vi "Init.vi"(5 "PathControl.lvclass":refnum<class "PathControl.lvclass">, 6 "Environmental classes":refnum<class "Instrument.lvclass">[](array[class]), 7 "XML Handler.lvclass":refnum<class "XML Handler.lvclass">, 8 "error in (no error)":errorcluster, 9 "Instrumentes to Use":T2(array[cluster]), 10 "Device.lvclass":refnum<class "Device.lvclass">, 11 "S Parameter in":refnum<class "S Parameter.lvclass">) -> (0 "error out":errorcluster, 3 "S Parameter out":refnum<class "S Parameter.lvclass">)   [LabVIEW 2020, in "S Parameter.lvclass"]
doc: "Initializes the measurement.\nThis verifies that the instruments are present and adds them into the class data.\nIs also adds the xml handler into the class data."
uses:
  S Parameter.lvclass
  Devices/Device.lvclass
  Instruments/Instrument.lvclass
  XML Handler/XML Handler.lvclass
  Path Control/PathControl.lvclass
  Controls/Init State Machine.ctl
  Instruments/Vector Network Analyzer/Vector Network Analyzer.lvclass
  S Parameter.lvclass/S Parameter.ctl
  Instruments/Vector Network Analyzer/Controls/S parm format enum.ctl
  Measurement.lvclass
panel:
  in  "S parameter":T1(ring)
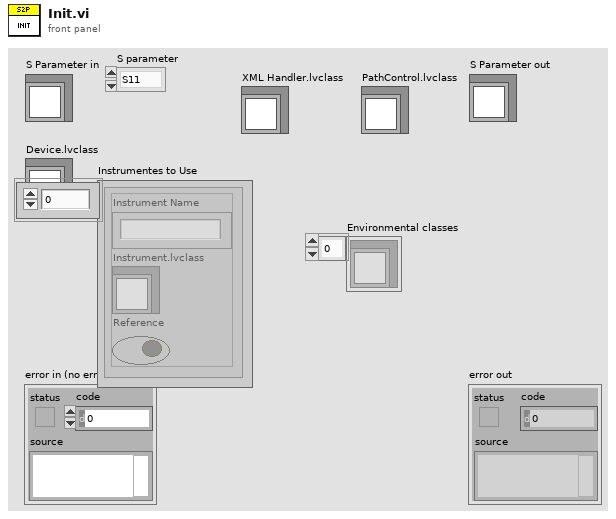
[diagram p1: front panel]
types:
  T1 = enum16{"S11", "S21", "S31", "S41", "S22", "S12", "S32", "S42", "S33", "S13", "S23", "S43", "S44", "S14", "S24", "S34"}
  T2 = cluster{"Instrument Name":string, "Instrument.lvclass":refnum<class "Instrument.lvclass">, "Reference":bool}[]
  T3 = typedef "S Parameter.lvclass/Init State Machine.ctl" = enum16{"Verify Instruments", "Init Instruments", "Init Device", "Create test in XML", "Set Path", "Done"}
  T4 = typedef "Vector Network Analyzer.lvclass/S parm format enum.ctl" = enum16{"Mag dB", "Mag", "Phase", "Smith", "Real", "Imag", "Group Delay", "SWR"}
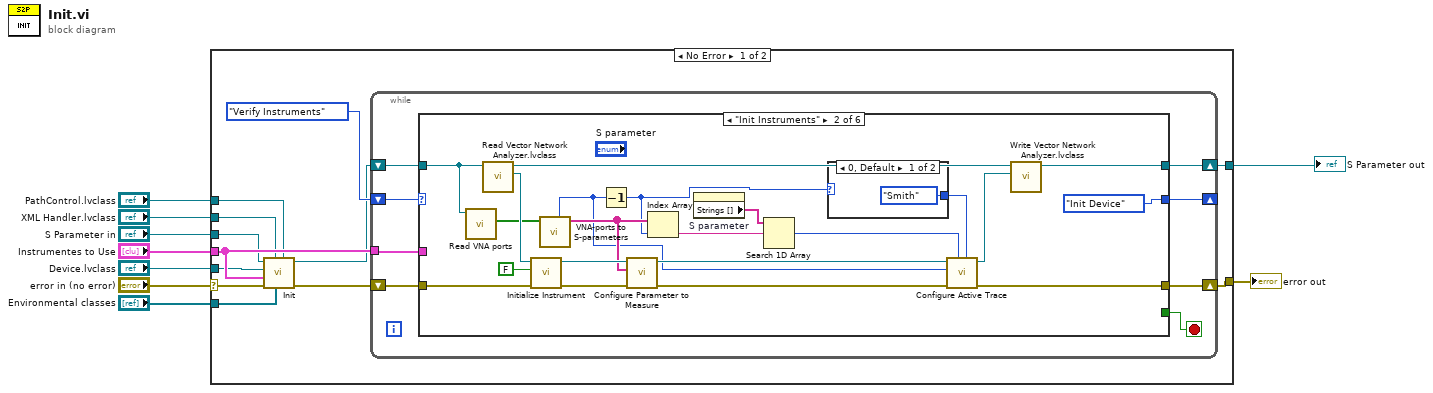
[diagram p0: block diagram]
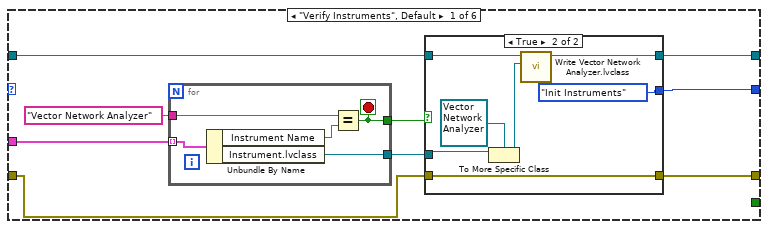
[diagram p2: hidden frame]
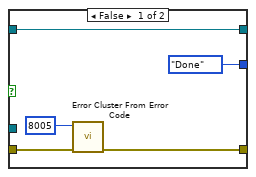
[diagram p3: hidden frame]
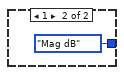
[diagram p4: hidden frame]
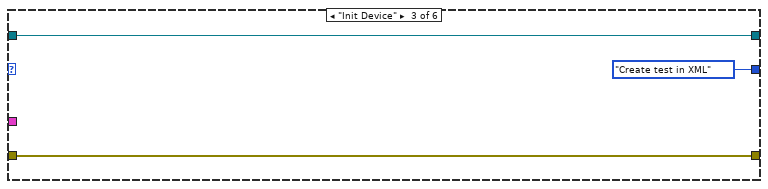
[diagram p5: hidden frame]
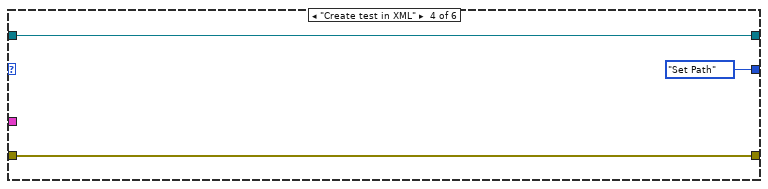
[diagram p6: hidden frame]
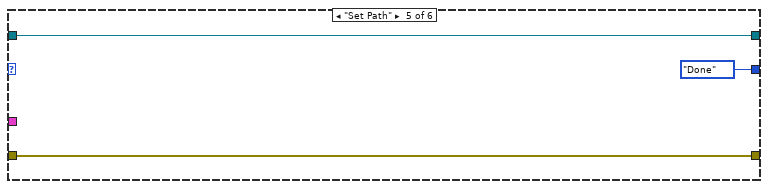
[diagram p7: hidden frame]
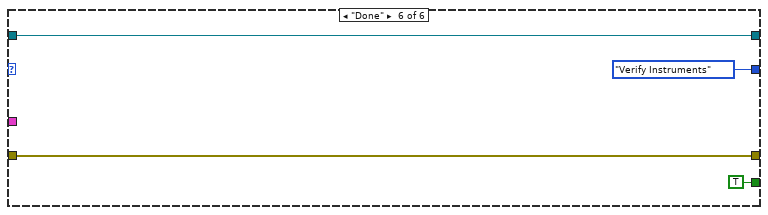
[diagram p8: hidden frame]
diagram:
  n1 = case shown="No Error" "error in (no error)" {
    selector: "error in (no error)" -> [w18 w92]
    tunnel: "S Parameter in" -> [w12 w93]
    tunnel: "Instrumentes to Use" -> [w15 _]
    tunnel: [w21 w93] -> w6
    tunnel: [w19 w92] -> w5
    tunnel: "Environmental classes" -> [w16 _]
    tunnel: "Device.lvclass" -> [w14 _]
    tunnel: "XML Handler.lvclass" -> [w13 _]
    tunnel: "PathControl.lvclass" -> [w10 _]
    frame No Error {
      n2 = call-parent "Init.vi"("PathControl.lvclass"=w10, "Environmental classes"=w16, "XML Handler.lvclass"=w13, "error in (no error)"=w18, "Instruments to Use"=w15, "Device.lvclass"=w14, "Measurements in"=w12) -> ("error out"=w17:errorcluster, "Measurements out"=w11:refnum<class "S Parameter.lvclass">)  [unwired: 3 in]
      n3 = while {
        tunnel: w15 -> [w29]
        shift-right: [w27] -> w21
        shift-left: w11 -> [w28]
        shift-right: [w25] -> _
        shift-left: Init_State_Machine."Verify Instruments" -> [w26]
        shift-right: [w23] -> w19
        shift-left: w17 -> [w24]
        stop <- w22 stop-if-true
        n4 = case shown="\"Init Instruments\"" w26 {
          tunnel: w29 -> [w38 _ _ _ _ _]
          tunnel: w28 -> [w35 w63 w80 w83 w87 w91]
          tunnel: [w33 w66 w80 w83 w87 w91] -> w27
          tunnel: [w30 Init_State_Machine."Init Device" Init_State_Machine."Create test in XML" Init_State_Machine."Set Path" Init_State_Machine."Done" Init_State_Machine."Verify Instruments"] -> w25
          tunnel: w24 -> [w32 w76 w81 w84 w85 w90]
          tunnel: [w31 w65 w81 w84 w85 w90] -> w23
          tunnel: [_ _ _ _ _ TRUE] -> w22
          frame "Verify Instruments", Default {
            n5 = for {
              tunnel: w38 -> [w55] mode=indexing
              tunnel: "Vector Network Analyzer" -> [w53]
              tunnel: [w52] -> w36
              tunnel: [w51] -> w34
              stop <- w52 stop-if-true
              n6 = Unbundle By Name(w55) -> ("Instrument Name"=w54:string, "Instrument.lvclass"=w51:refnum<class "Instrument.lvclass">)
              n7 = Equal?(x=w53, y=w54) -> (x = y?=w52:bool)
            }
            n8 = case shown="True" w36 {
              tunnel: w35 -> [w43 w50]
              tunnel: w34 -> [_ w48]
              tunnel: [w43 w49] -> w33
              tunnel: w32 -> [w42 w45]
              tunnel: [w40 w45] -> w31
              tunnel: [Init_State_Machine."Done" Init_State_Machine."Init Instruments"] -> w30
              frame False {
                n9 = call <vilib>:"Error Cluster From Error Code.vi"("error in (no error)"=w42, "error code (0)"=8005) -> ("error out"=w40:errorcluster)  [unwired: 7 in]
              }
              frame True {
                n10 = To More Specific Class(target class=refnum<class "Vector Network Analyzer.lvclass"> refnum ("Vector Network Analyzer.lvclass"), reference=w48) -> (specific class reference=w46:refnum<class "Vector Network Analyzer.lvclass">)  [unwired: 1 in, 1 out]
                n11 = call "Write Vector Network Analyzer.lvclass.vi"("Vector Network Analyzer.lvclass"=w46, "S Parameter in"=w50) -> ("S Parameter out"=w49:refnum<class "S Parameter.lvclass">)  [unwired: 9 in]
              }
            }
          }
          frame "Init Instruments" {
            n12 = call-dynamic "Read VNA ports.vi"("S Parameter in"=w63) -> ("VNA ports"=w62:bool[])  [unwired: 9 in, 1 out]
            n13 = call "Read Vector Network Analyzer.lvclass.vi"("S Parameter in"=w63) -> ("Vector Network Analyzer.lvclass"=w75:refnum<class "Vector Network Analyzer.lvclass">, "S Parameter out"=w73:refnum<class "S Parameter.lvclass">)  [unwired: 9 in]
            n14 = call-dynamic "Initialize Instrument.vi"("error in (no error)"=w76, "Reset"=FALSE, "Instrument in"=w75) -> ("error out"=w72:errorcluster, "Instrument out"=w71:refnum<class "Vector Network Analyzer.lvclass">)  [unwired: 7 in]
            n15 = call "VNA-ports to S-parameters.vi"("VNA ports"=w62) -> ("Sparameters (string)"=w58:string[], "Number of ports"=w56:i32)  [unwired: 6 in, 3 out]
            n16 = Decrement(x=w56) -> (x-1=w57:i32)
            n17 = call-dynamic "Configure Parameter to Measure.vi"("error in (no error)"=w72, "Sparameters (string)"=w58, "Vector Network Analyzer in"=w71) -> ("error out"=w70:errorcluster, "Vector Network Analyzer out"=w69:refnum<class "Vector Network Analyzer.lvclass">)  [unwired: 7 in]
            n18 = Index Array(array=w58, index=w57) -> (element=w60:string)
            n19 = property on="S parameter" class="Enum (strict)"() -> ("Strings []"=w61:string[])  [unwired: 2 in, 2 out]
            n20 = Search 1D Array(1D array=w61, element=w60) -> (index of element=w59:i32)  [unwired: 1 in]
            n21 = case shown="0, Default" w57 {
              tunnel: [S_parm_format_enum."Smith" ("Format") S_parm_format_enum."Mag dB" ("Format")] -> w68
              frame 0, Default {
              }
              frame 1 {
              }
            }
            n22 = call-dynamic "Configure Active Trace.vi"("Format"=w68, "S parameter"=w59, "error in (no error)"=w70, "Active Trace"=w56, "Vector Network Analyzer in"=w69) -> ("error out"=w65:errorcluster, "Vector Network Analyzer out"=w67:refnum<class "Vector Network Analyzer.lvclass">)  [unwired: 5 in]
            n23 = call "Write Vector Network Analyzer.lvclass.vi"("Vector Network Analyzer.lvclass"=w67, "S Parameter in"=w73) -> ("S Parameter out"=w66:refnum<class "S Parameter.lvclass">)  [unwired: 9 in]
          }
          frame "Init Device" {
          }
          frame "Create test in XML" {
          }
          frame "Set Path" {
          }
          frame "Done" {
          }
        }
      }
    }
    frame Error {
    }
  }
  "error out" <- w5
  "S Parameter out" <- w6
